vi "MultiChannelFeedbackCooling(Host).vi"(5 "RIO Device":T1="RIO0::INSTR") -> ()   [LabVIEW 2013]
doc: "This VI will will initialize the FPGA VI and then continually read and convert single point values from 4 channels of an analog input module."
uses:
  <vilib>/userdefined/High Color/nirio_resource_hc.ctl
  <vilib>/FPGAPlugInAG/PCIe-7841R/niLvFpga_Open_PCIe-7841R.vi
  <vilib>/FPGAPlugInAG/PCIe-7841R/niLvFpga_Run_PCIe-7841R.vi
  <vilib>/Utility/error.llb/Error Cluster From Error Code.vi
  <vilib>/rvi/errors/niLvFpgaAdjustHostInterfaceError.vi
  <vilib>/Utility/file.llb/Read From Spreadsheet File (I64).vi
  <vilib>/FPGAPlugInAG/PCIe-7841R/niLvFpga_Close_PCIe-7841R.vi
  <vilib>/rvi/interface/nirviOpenFPGA/nirviOpenFPGA.xnode
  FPGA Bitfiles/MultiChannelFeed_FPGATarget2_MultiChannelfFee_lERQoxjCHp8.lvbitx
  <vilib>/rvi/interface/nirviMethod/nirviMethod.xnode
  <vilib>/rvi/interface/nirviReadWriteControl/nirviReadWriteControl.xnode
  <vilib>/rvi/interface/nirviCloseFPGA/nirviCloseFPGA.xnode
  NiFpgaLv.dll
panel:
  in  "ramp arb drive":bool
  in  "End value arb":fxp<+/-,32,16>
  in  "Step arb":fxp<+/-,32,16>
  in  "Delay Time (s) arb":dbl caption="Delay Time (s)"
  in  "Buffer file path":path=path "D:/GitHub/opt_lev/labview/fpga/triangle_buffer.txt"
  in  "Write data to buffers":bool
  in  "Arb steps per cycle":u16
  in  "Arb gain (ch2)":fxp<+,32,16>
  in  "Arb gain (ch1)":fxp<+,32,16>
  in  "meters per measured bit 0":fxp<+/-,32,16>=1.0
  in  "meters per measured bit 1":fxp<+/-,32,16>=1.0
  in  "apply corrections":bool
  in  "ramp drive 1":bool
  in  "End value 2":fxp<+/-,32,16>
  in  "Step 2":fxp<+/-,32,16>=1.52587890625e-05
  in  "Delay Time (s) 2":dbl=0.01 caption="Delay Time (s)"
  in  "ramp drive 0":bool
  in  "End value":fxp<+/-,32,16>
  in  "Step":fxp<+/-,32,16>
  in  "Delay Time (s)":dbl
  out "feedback + dc 2":i16(graph)=9000
  out "feedback +dc +drive 1":i16(graph)=14000
  out "feedback + dc + drive 0":i16(graph)=15500
  out "feedback only 1":dbl(graph)
  out "feedback only 0":i16(graph)
  out "AI1":i16(graph)=8089
  out "AI1":i16(graph)=-1105
  in  "Z offset 1":fxp<+/-,32,16>=1.0
  in  "Z offset 0":fxp<+/-,32,16>=1.0
  in  "Zfb norm const 1":fxp<+/-,32,16>=1.0
  in  "Zfb norm const 0":fxp<+/-,32,16>=1.0
  in  "Dc Pos 1":fxp<+/-,32,16>=1.0
  in  "Dc Pos 0":fxp<+/-,32,16>=1.0
  in  "meters per bit beam displacement 1":fxp<+/-,32,16>=1.0
  in  "meters per bit beam displacement 0":fxp<+/-,32,16>=1.0
  in  "Drive_gain 1":fxp<+/-,32,16>
  in  "Drive_gain 0":fxp<+/-,32,16>
  in  "frequency (periods/tick)":fxp<+,32,0>=5.005858838558197e-08
  in  "change pars 2":bool
  in  "3, 1":fxp<+/-,32,16>
  in  "3, 2":fxp<+/-,32,16>
  in  "3, 3":fxp<+/-,32,16>=1.0
  in  "2, 3":fxp<+/-,32,16>
  in  "2, 2":fxp<+/-,32,16>=1.0
  in  "2, 1":fxp<+/-,32,16>
  in  "1, 3":fxp<+/-,32,16>
  in  "1, 2":fxp<+/-,32,16>
  in  "1,1":fxp<+/-,32,16>=1.0
  out "AI0":i16(graph)=-1504
  in  "Dc offset 2":fxp<+/-,32,16>=9000.0
  in  "Lower lim 2":fxp<+/-,32,16>=-3000.0
  in  "Upper lim 2":fxp<+/-,32,16>=3000.0
  in  "dg 2":fxp<+/-,32,16>
  in  "pg 2":fxp<+/-,32,16>
  in  "Setpoint 2":fxp<+/-,32,16>
  in  "Dc offset 1":fxp<+/-,32,16>=14000.0
  in  "Upper lim 1":fxp<+/-,32,16>=3600.0
  in  "Lower lim 1":fxp<+/-,32,16>=-3600.0
  in  "dg 1":fxp<+/-,32,16>
  in  "pg 1":fxp<+/-,32,16>
  in  "Dc offset 0":fxp<+/-,32,16>=15500.0
  in  "Lower lim 0":fxp<+/-,32,16>=-2000.0
  in  "Upper lim 0":fxp<+/-,32,16>=2000.0
  in  "dg 0":fxp<+/-,32,16>
  in  "pg 0":fxp<+/-,32,16>
  in  "Setpoint 0":fxp<+/-,32,16>=1.0
  in  "change pars":bool
  in  "stop":bool
  # "Analog Input"
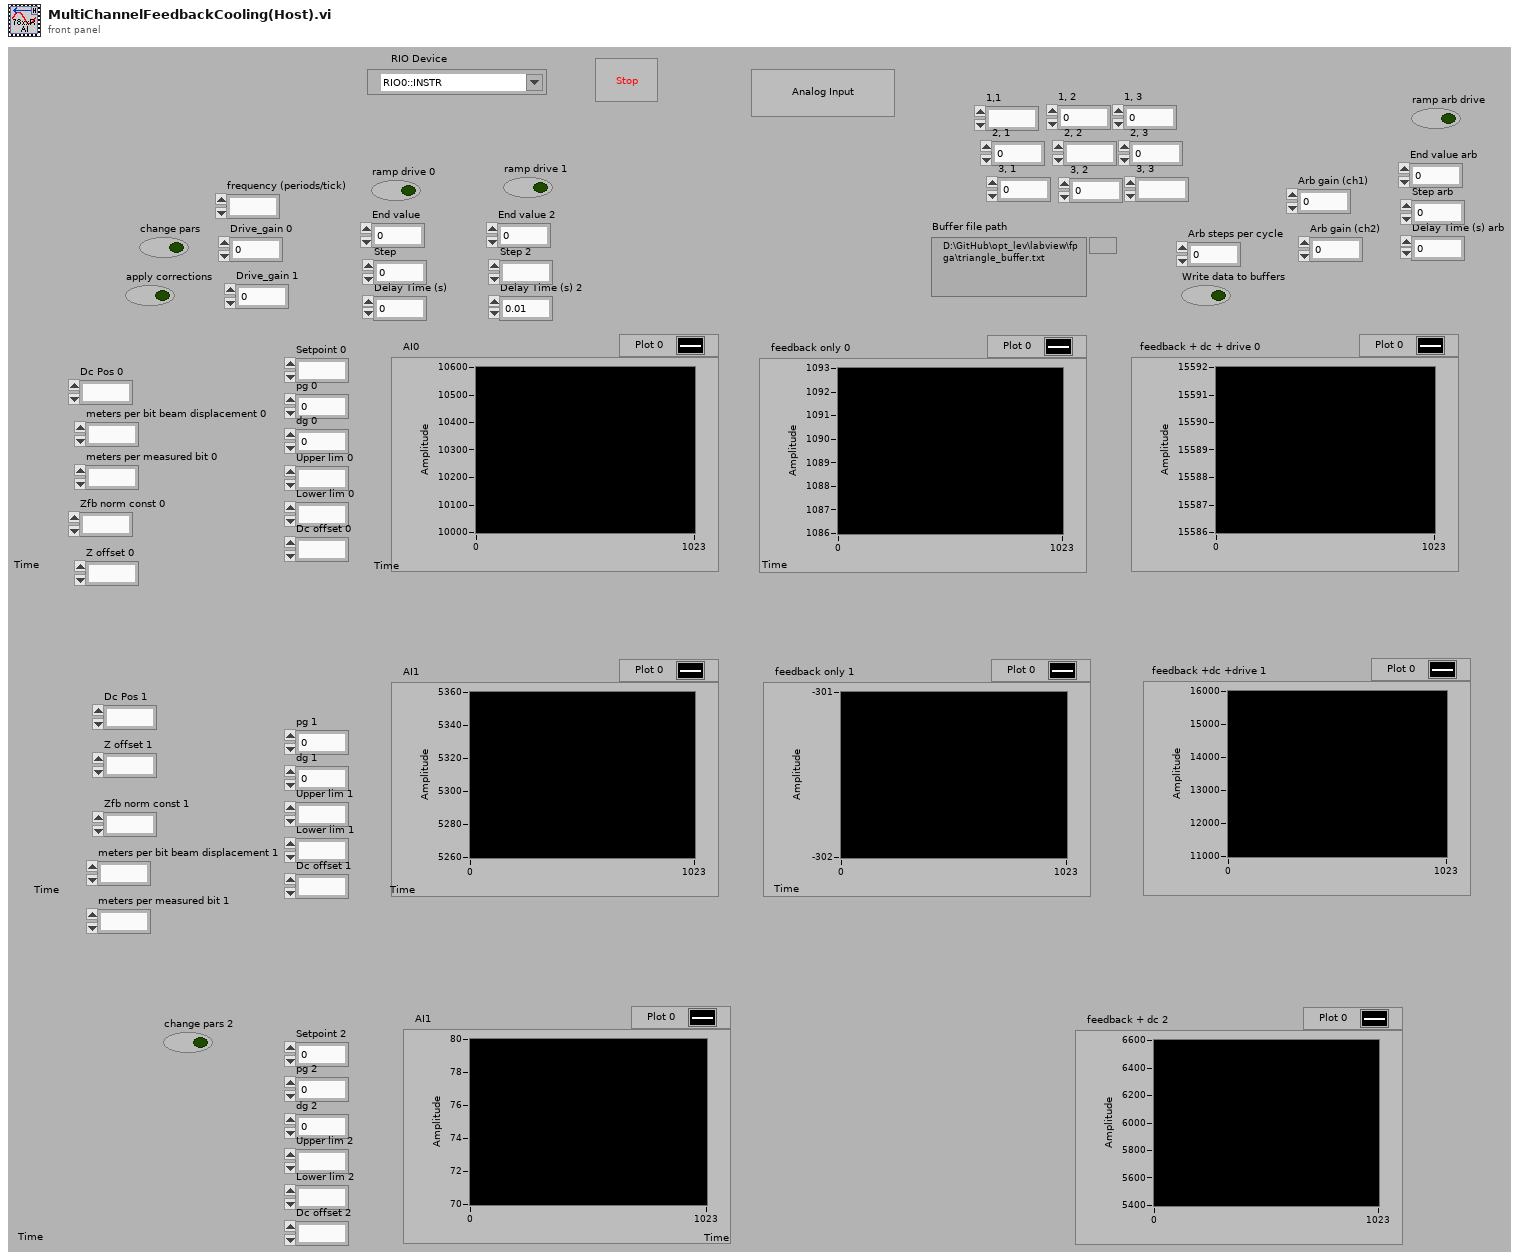
[diagram p1: front panel]
types:
  T1 = typedef "nirio_resource_hc.ctl" = tag
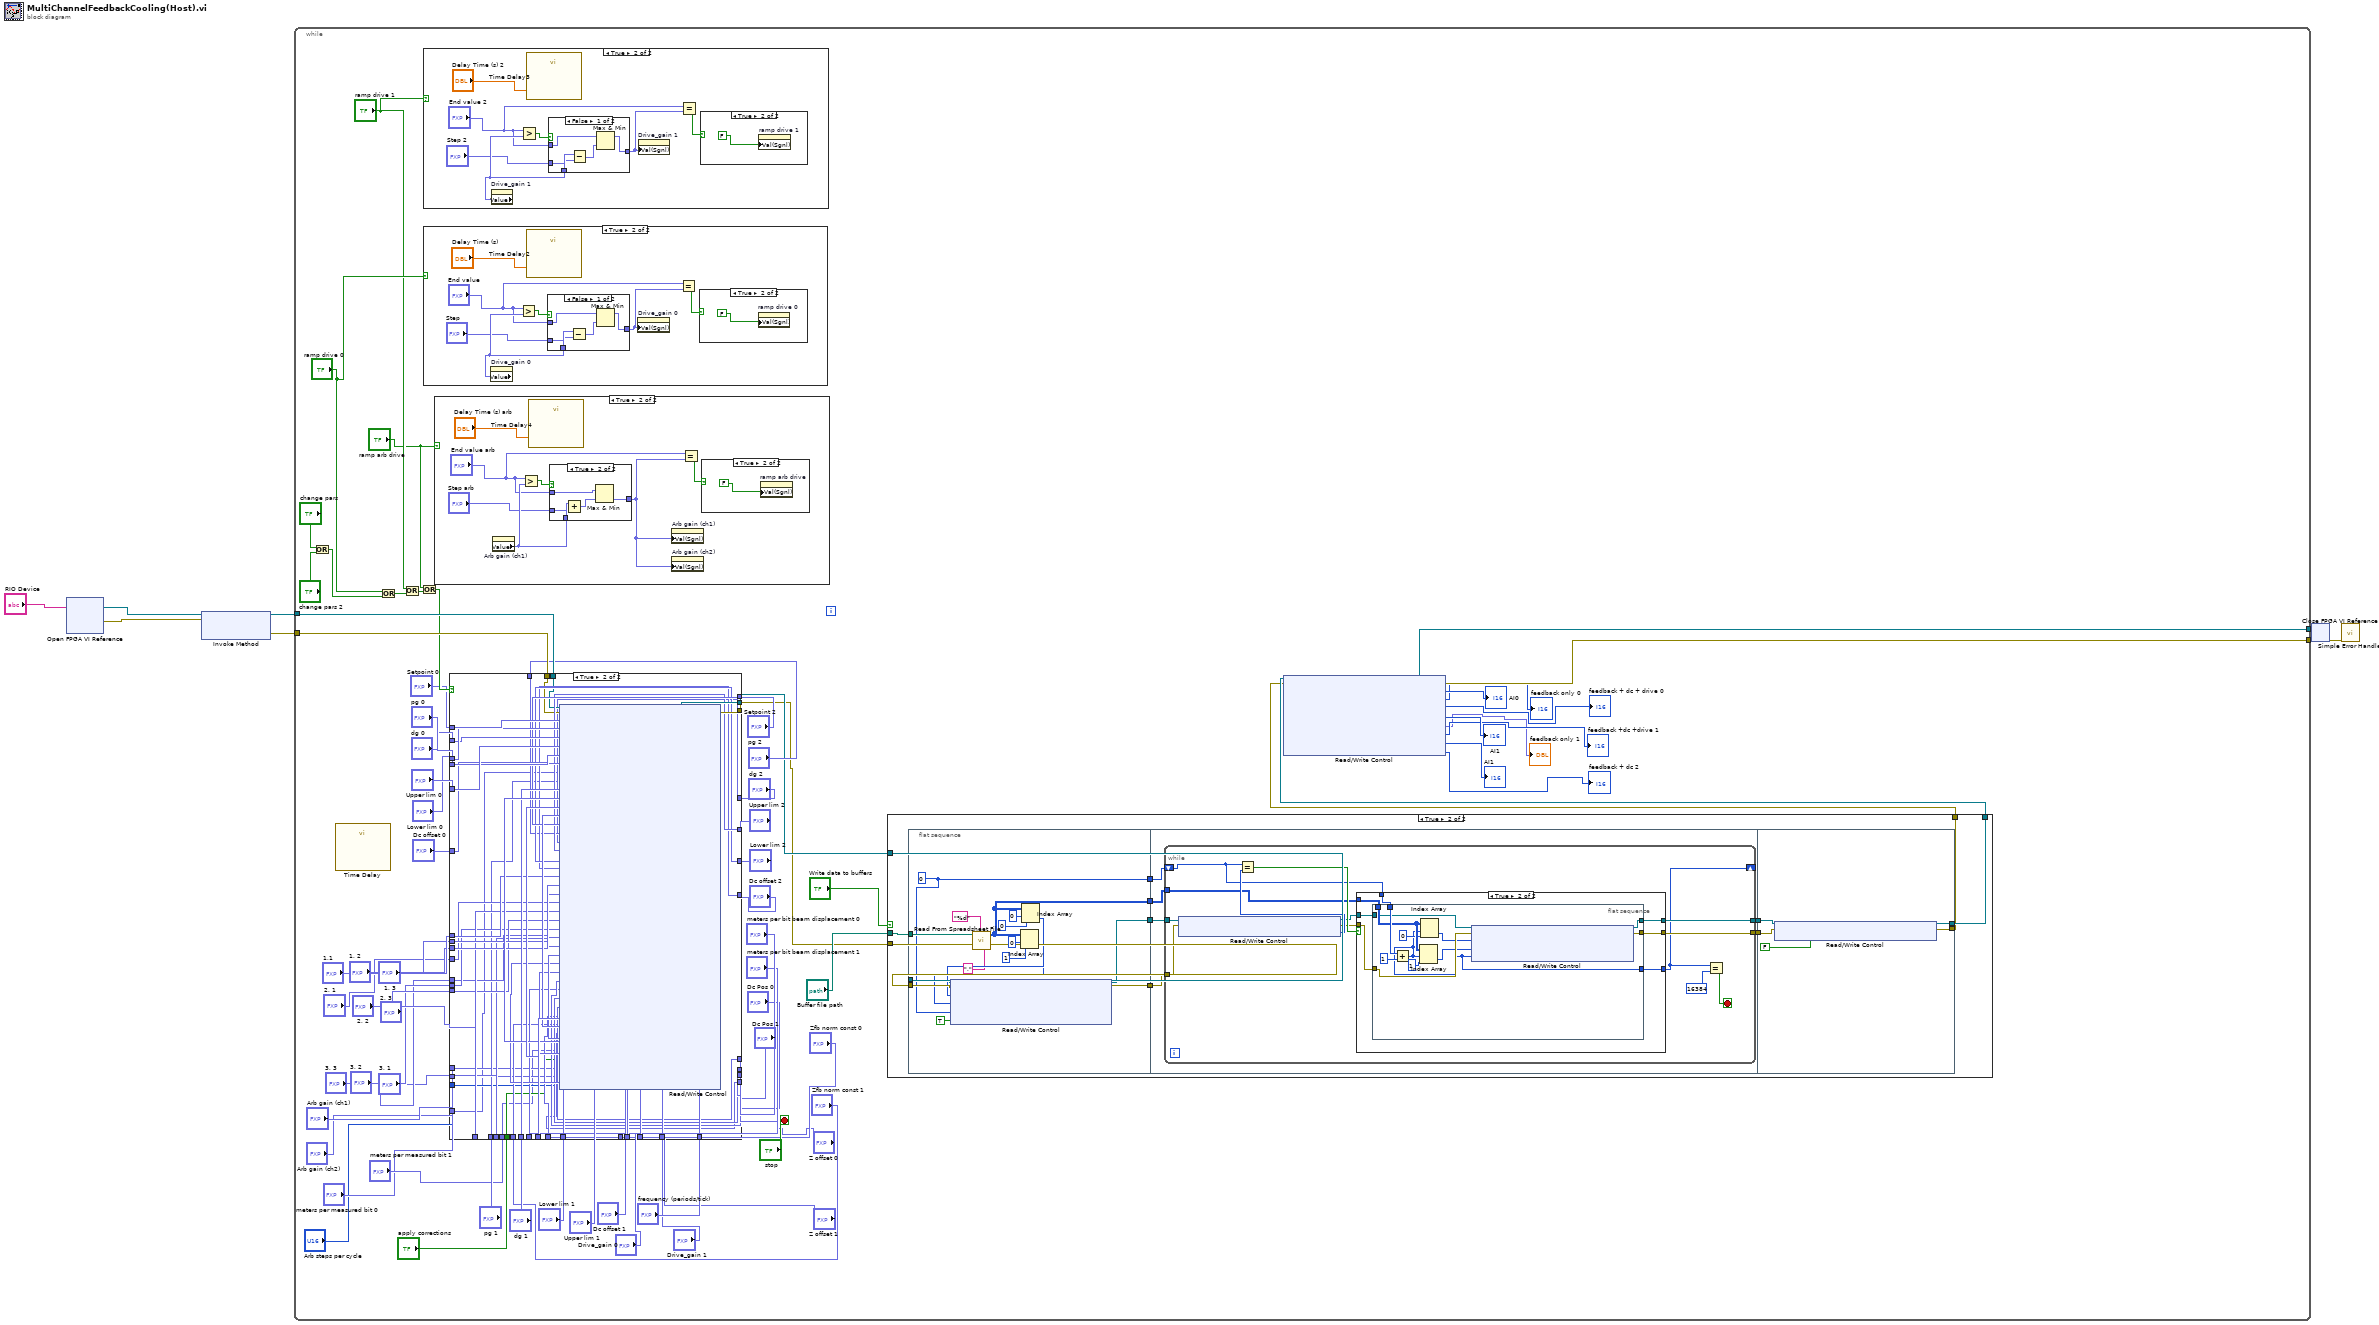
[diagram p0: block diagram]
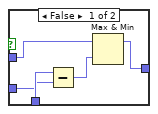
[diagram p4: hidden frame]
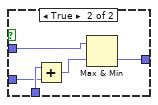
[diagram p9: hidden frame]
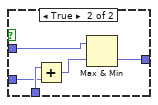
[diagram p12: hidden frame]
diagram:
  n1 = xnode "Open FPGA VI Reference"("resource name"="RIO Device") -> ("FPGA VI Reference Out"=w3:refnum<k20>, "error out"=w2:errorcluster)  [unwired: 1 in]
  n2 = xnode "Invoke Method"("FPGA VI Reference In"=w3, "error in"=w2) -> ("FPGA VI Reference Out"=w5:refnum<k20>, "error out"=w4:errorcluster)  [unwired: 1 in]
  n3 = while {
    tunnel: [w79] -> w8
    tunnel: w5 -> [w51]
    tunnel: w4 -> [w50]
    tunnel: [w78] -> w1
    stop <- "stop" stop-if-true
    n4 = Or(x="change pars", y="change pars 2") -> (x .or. y?=w32:bool)
    n5 = call "Time Delay"() -> ()  [unwired: 11 in, 1 out]
    n6 = Or(x="ramp drive 0", y=w32) -> (x .or. y?=w30:bool)
    n7 = Or(x="ramp drive 1", y=w30) -> (x .or. y?=w13:bool)
    n8 = Or(x="ramp arb drive", y=w13) -> (x .or. y?=w12:bool)
    n9 = case shown="True" "ramp drive 0" {
      frame False {
      }
      frame True {
        n10 = property on="Drive_gain 0" class="DigNum (strict)"() -> ("Value"=w196:fxp<+/-,32,16>)  [unwired: 2 in, 2 out]
        n11 = Greater?(x="End value", y=w196) -> (0:w197:bool)
        n12 = call "Time Delay2"("Delay Time (s)"="Delay Time (s)") -> ()  [unwired: 10 in, 1 out]
        n13 = case shown="False" w197 {
          tunnel: "End value" -> [w200 w205]
          tunnel: w196 -> [w203 w208]
          tunnel: "Step" -> [w202 w207]
          tunnel: [w199 w204] -> w195
          frame False {
            n14 = Subtract(x=w203, y=w202) -> (x-y=w201:fxp<+/-,33,17>)
            n15 = Max & Min(x=w200, y=w201) -> (max(x,y)=w199:fxp<+/-,33,17>)  [unwired: 1 out]
          }
          frame True {
            n16 = Add(x=w208, y=w207) -> (x+y=w206:fxp<+/-,33,17>)
            n17 = Max & Min(x=w205, y=w206) -> (min(x,y)=w204:fxp<+/-,33,17>)  [unwired: 1 out]
          }
        }
        n18 = property on="Drive_gain 0" class="DigNum (strict)"("Val(Sgnl)"=w195) -> ()  [unwired: 2 in, 2 out]
        n19 = Equal?(x="End value", y=w195) -> (x = y?=w194:bool)
        n20 = case shown="True" w194 {
          frame False {
          }
          frame True {
            n21 = property on="ramp drive 0" class="Bool (strict)"("Val(Sgnl)"=FALSE) -> ()  [unwired: 2 in, 2 out]
          }
        }
      }
    }
    n22 = case shown="True" "ramp drive 1" {
      frame False {
      }
      frame True {
        n23 = property on="Drive_gain 1" class="DigNum (strict)"() -> ("Value"=w178:fxp<+/-,32,16>)  [unwired: 2 in, 2 out]
        n24 = Greater?(x="End value 2", y=w178) -> (0:w179:bool)
        n25 = call "Time Delay3"("Delay Time (s)"="Delay Time (s) 2") -> ()  [unwired: 10 in, 1 out]
        n26 = case shown="False" w179 {
          tunnel: "End value 2" -> [w182 w187]
          tunnel: w178 -> [w185 w190]
          tunnel: "Step 2" -> [w184 w189]
          tunnel: [w181 w186] -> w177
          frame False {
            n27 = Subtract(x=w185, y=w184) -> (x-y=w183:fxp<+/-,33,17>)
            n28 = Max & Min(x=w182, y=w183) -> (max(x,y)=w181:fxp<+/-,33,17>)  [unwired: 1 out]
          }
          frame True {
            n29 = Add(x=w190, y=w189) -> (x+y=w188:fxp<+/-,33,17>)
            n30 = Max & Min(x=w187, y=w188) -> (min(x,y)=w186:fxp<+/-,33,17>)  [unwired: 1 out]
          }
        }
        n31 = property on="Drive_gain 1" class="DigNum (strict)"("Val(Sgnl)"=w177) -> ()  [unwired: 2 in, 2 out]
        n32 = Equal?(x="End value 2", y=w177) -> (x = y?=w176:bool)
        n33 = case shown="True" w176 {
          frame False {
          }
          frame True {
            n34 = property on="ramp drive 1" class="Bool (strict)"("Val(Sgnl)"=FALSE) -> ()  [unwired: 2 in, 2 out]
          }
        }
      }
    }
    n35 = case shown="True" "ramp arb drive" {
      frame False {
      }
      frame True {
        n36 = property on="Arb gain (ch1)" class="DigNum (strict)"() -> ("Value"=w85:fxp<+,32,16>)  [unwired: 2 in, 2 out]
        n37 = Greater?(x="End value arb", y=w85) -> (0:w86:bool)
        n38 = call "Time Delay4"("Delay Time (s)"="Delay Time (s) arb") -> ()  [unwired: 10 in, 1 out]
        n39 = case shown="True" w86 {
          tunnel: "End value arb" -> [w89 w94]
          tunnel: w85 -> [w92 w97]
          tunnel: "Step arb" -> [w91 w96]
          tunnel: [w88 w93] -> w80
          frame False {
            n40 = Subtract(x=w92, y=w91) -> (x-y=w90:fxp<+/-,34,18>)
            n41 = Max & Min(x=w89, y=w90) -> (max(x,y)=w88:fxp<+/-,34,18>)  [unwired: 1 out]
          }
          frame True {
            n42 = Add(x=w97, y=w96) -> (x+y=w95:fxp<+/-,34,18>)
            n43 = Max & Min(x=w94, y=w95) -> (min(x,y)=w93:fxp<+/-,34,18>)  [unwired: 1 out]
          }
        }
        n44 = property on="Arb gain (ch1)" class="DigNum (strict)"("Val(Sgnl)"=w80) -> ()  [unwired: 2 in, 2 out]
        n45 = property on="Arb gain (ch2)" class="DigNum (strict)"("Val(Sgnl)"=w80) -> ()  [unwired: 2 in, 2 out]
        n46 = Equal?(x="End value arb", y=w80) -> (x = y?=w84:bool)
        n47 = case shown="True" w84 {
          frame False {
          }
          frame True {
            n48 = property on="ramp arb drive" class="Bool (strict)"("Val(Sgnl)"=FALSE) -> ()  [unwired: 2 in, 2 out]
          }
        }
      }
    }
    n49 = case shown="True" w12 {
      tunnel: w50 -> [w210 w231]
      tunnel: [w210 w257] -> w16
      tunnel: [w209 w256] -> w17
      tunnel: "Setpoint 0" -> [_ w255]
      tunnel: "pg 0" -> [_ w254]
      tunnel: "dg 0" -> [_ w253]
      tunnel: "Upper lim 0" -> [_ w252]
      tunnel: "Lower lim 0" -> [_ w251]
      tunnel: "Dc offset 0" -> [_ w250]
      tunnel: "Dc offset 1" -> [_ w249]
      tunnel: "Upper lim 1" -> [_ w248]
      tunnel: "Lower lim 1" -> [_ w247]
      tunnel: "dg 1" -> [_ w246]
      tunnel: "Setpoint 2" -> [_ w245]
      tunnel: "Upper lim 2" -> [_ w244]
      tunnel: "Lower lim 2" -> [_ w243]
      tunnel: "Dc offset 2" -> [_ w242]
      tunnel: "1,1" -> [_ w241]
      tunnel: "1, 2" -> [_ w240]
      tunnel: "1, 3" -> [_ w239]
      tunnel: "2, 1" -> [_ w238]
      tunnel: "2, 2" -> [_ w237]
      tunnel: "2, 3" -> [_ w236]
      tunnel: "3, 3" -> [_ w235]
      tunnel: "3, 2" -> [_ w234]
      tunnel: "3, 1" -> [_ w233]
      tunnel: w51 -> [w209 w230]
      tunnel: "frequency (periods/tick)" -> [_ w232]
      tunnel: "Drive_gain 0" -> [_ w229]
      tunnel: "Drive_gain 1" -> [_ w228]
      tunnel: "meters per bit beam displacement 0" -> [_ w227]
      tunnel: "meters per bit beam displacement 1" -> [_ w226]
      tunnel: "Dc Pos 0" -> [_ w225]
      tunnel: "Dc Pos 1" -> [_ w224]
      tunnel: "Zfb norm const 0" -> [_ w223]
      tunnel: "Zfb norm const 1" -> [_ w222]
      tunnel: "Z offset 0" -> [_ w221]
      tunnel: "Z offset 1" -> [_ w220]
      tunnel: "pg 2" -> [_ w219]
      tunnel: "dg 2" -> [_ w218]
      tunnel: "pg 1" -> [_ w217]
      tunnel: "apply corrections" -> [_ w212]
      tunnel: "meters per measured bit 1" -> [_ w211]
      tunnel: "meters per measured bit 0" -> [_ w213]
      tunnel: "Arb gain (ch1)" -> [_ w216]
      tunnel: "Arb gain (ch2)" -> [_ w215]
      tunnel: "Arb steps per cycle" -> [_ w214]
      frame False {
      }
      frame True {
        n50 = xnode "Read/Write Control"("FPGA VI Reference In"=w230, "error in"=w231, "Dc Pos 0"=w255, "pg 0"=w254, "dg 0"=w253, "Upper lim 0"=w252, "Lower lim 0"=w251, "Dc offset 0"=w250, "meters per measured bit 0"=w213, "pg 1"=w217, "dg 1"=w246, "Lower lim 1"=w247, "Upper lim 1"=w248, "Dc offset 1"=w249, "Dc Pos 2"=w245, "pg 2"=w219, "dg 2"=w218, "Upper lim 2"=w244, "Lower lim 2"=w243, "Dc offset 2"=w242, "1,1"=w241, "1, 2"=w240, "1, 3"=w239, "2, 1"=w238, "2, 2"=w237, "2, 3"=w236, "3, 3"=w235, "3, 2"=w234, "3, 1"=w233, "frequency (periods/tick)"=w232, "Drive_gain 0"=w229, "Drive_gain 1"=w228, "meters per bit beam displacement 0"=w227, "meters per bit beam displacement 1"=w226, "Dc Pos 0"=w225, "Dc Pos 1"=w224, "Zfb norm const 0"=w223, "Zfb norm const"=w222, "Z offset 0"=w221, "Z offset 1"=w220, "meters per measured bit 1"=w211, "apply corrections"=w212, "Arb gain (ch1)"=w216, "Arb gain (ch2)"=w215, "Arb steps per cycle"=w214) -> ("FPGA VI Reference Out"=w256:refnum<k20>, "error out"=w257:errorcluster)
      }
    }
    n51 = case shown="True" "Write data to buffers" {
      tunnel: "Buffer file path" -> [_ w110]
      tunnel: w17 -> [w99 w109]
      tunnel: w16 -> [w98 w108]
      tunnel: [w99 w101] -> w15
      tunnel: [w98 w100] -> w14
      frame False {
      }
      frame True {
        n52 = flat-sequence {
          tunnel: w110 -> [w126]
          tunnel: w109 -> [w124]
          tunnel: w108 -> [w123]
          tunnel: [w118] -> w107
          tunnel: [w117] -> w106
          tunnel: [w116] -> w105
          tunnel: [w115] -> w104
          tunnel: w107 -> [w132]
          tunnel: w106 -> [w131]
          tunnel: w105 -> [w130]
          tunnel: w104 -> [w129]
          tunnel: [w128] -> w103
          tunnel: [w127] -> w102
          tunnel: w103 -> [w172]
          tunnel: w102 -> [w171]
          tunnel: [w170] -> w101
          tunnel: [w169] -> w100
          frame #0 {
            w115 = 0
            n53 = call-poly <vilib>:"Read From Spreadsheet File.vi"("delimiter (\\t)"="," ("delimiter (\\t)"), "format (%d)"="%d", "file path (dialog if empty)"=w126) -> ("all rows"=w116:i64[][])  [unwired: 4 in, 4 out]
            n54 = Index Array(array=w116, index (row)=0, index (col)=1 ("disabled index (col)")) -> (element=w114:i64)
            n55 = Index Array(array=w116, index (row)=0, index (col)=0 ("disabled index (col)")) -> (element=w113:i64)
            n56 = xnode "Read/Write Control"("FPGA VI Reference In"=w124, "error in"=w123, "data_buffer_1"=w114, "data_buffer2"=w113, "write_address"=w115, "ready_to_write"=TRUE) -> ("FPGA VI Reference Out"=w117:refnum<k20>, "error out"=w118:errorcluster)
          }
          frame #1 {
            n57 = while {
              shift-right: [w133] -> _
              shift-left: w129 -> [w141]
              tunnel: w131 -> [w145]
              tunnel: w132 -> [w144]
              tunnel: w130 -> [w140]
              tunnel: [w135] -> w128
              tunnel: [w134] -> w127
              stop <- w136 stop-if-true
              n58 = xnode "Read/Write Control"("FPGA VI Reference In"=w145, "error in"=w144) -> ("FPGA VI Reference Out"=w139:refnum<k20>, "error out"=w138:errorcluster, "written_address"=w143:u32)
              n59 = Equal?(x=w141, y=w143) -> (x = y?=w142:bool)
              n60 = case shown="True" w142 {
                tunnel: w141 -> [w148 w155]
                tunnel: w140 -> [_ w154]
                tunnel: w139 -> [w147 w153]
                tunnel: w138 -> [w146 w152]
                tunnel: [w148 w151] -> w133
                tunnel: [w147 w150] -> w135
                tunnel: [w146 w149] -> w134
                frame False {
                }
                frame True {
                  n61 = flat-sequence {
                    tunnel: w155 -> [w166]
                    tunnel: w154 -> [w165]
                    tunnel: w153 -> [w162]
                    tunnel: w152 -> [w161]
                    tunnel: [w157] -> w151
                    tunnel: [w159] -> w150
                    tunnel: [w158] -> w149
                    frame #0 {
                      n62 = Add(x=w166, y=1) -> (x+y=w157:i32)
                      n63 = Index Array(array=w165, index (row)=w157, index (col)=1 ("disabled index (col)")) -> (element=w160:i64)
                      n64 = Index Array(array=w165, index (row)=w157, index (col)=0 ("disabled index (col)")) -> (element=w156:i64)
                      n65 = xnode "Read/Write Control"("FPGA VI Reference In"=w162, "error in"=w161, "data_buffer_1"=w156, "data_buffer2"=w160, "write_address"=w157) -> ("FPGA VI Reference Out"=w159:refnum<k20>, "error out"=w158:errorcluster)
                    }
                  }
                }
              }
              n66 = Equal?(x=w133, y=u16 16384) -> (x = y?=w136:bool)
            }
          }
          frame #2 {
            n67 = xnode "Read/Write Control"("FPGA VI Reference In"=w172, "error in"=w171, "ready_to_write"=FALSE) -> ("FPGA VI Reference Out"=w170:refnum<k20>, "error out"=w169:errorcluster)
          }
        }
      }
    }
    n68 = xnode "Read/Write Control"("FPGA VI Reference In"=w15, "error in"=w14) -> ("FPGA VI Reference Out"=w79:refnum<k20>, "error out"=w78:errorcluster, "AI0"=→"AI0":i16, "fb_0"=→"feedback only 0":i16, "fb+dc+drive_0"=→"feedback + dc + drive 0":i16, "Connector0/AI1"=→"AI1":i16, "fb_1"=→"feedback only 1":fxp<+/-,16,16>, "fb+dc+drive_1"=→"feedback +dc +drive 1":i16, "Connector0/AI2"=→"AI1":i16, "fb +dc_2"=→"feedback + dc 2":i16)
  }
  n69 = xnode "Close FPGA VI Reference"("FPGA VI Reference In"=w8, "error in"=w1) -> ("error out"=w7:errorcluster)
  n70 = call <vilib>:"Simple Error Handler.vi"("error in (no error)"=w7) -> ()  [unwired: 4 in, 5 out]
